vi "Streaming 2945 2955 (FPGA).vi"() -> ()   [LabVIEW 2016]
doc: "Acquires data from the Rx ports and streams the data to the host while receiving data from the host and generating the resulting waveform at the Tx ports of the NI USRP 294x/295x device. Use this VI as a template for the Simple NI-USRP Streaming sample project."
uses:
  <instrlib>/_niInstr/Register Bus/v1/FPGA/Public/Read Cmd Data.ctl
  SubVIs/Stream Control State.ctl
  SubVIs/Rx Parameters.ctl
  HOST/29x5/SubVIs/Start Trigger.ctl
  SubVIs/DDC Parameters.ctl
  <instrlib>/_niInstr/DSP/v1/Shared/Public/IQ Impairments.ctl
  <instrlib>/_niInstr/DSP/v1/Shared/Public/IQ Gain.ctl
  <vilib>/Platform/TimedLoop/XDataNode/timing_clust.ctl
  <vilib>/Platform/TimedLoop/XDataNode/nitl_modes.ctl
  <vilib>/Platform/TimedLoop/XDataNode/wakeup.ctl
  SubVIs/Tx Parameters.ctl
  SubVIs/DUC Parameters.ctl
  <vilib>/rvi/Emulation/niFpgaSctlEmulationGetInTimedLoop.vi
  <vilib>/rvi/Emulation/niFpgaEmulationReportErrorSimple.vi
  <vilib>/rvi/Emulation/niFpgaGetClockAttributes.vi
  <vilib>/rvi/Emulation/niFpgaCriticalErrorInLSC.vi
  <vilib>/rvi/Emulation/niFpgaProcessEmulError.vi
  <vilib>/rvi/Emulation/niFpgaEmulationIsFPGAContextNoSignature.vi
  <vilib>/rvi/DataTransferAndStorage/Container/Common/niFpgaContainerGetUniqueNameForEmu.vi
  <vilib>/rvi/Memory/Memory_Emulation/niFpgaMemoryEmulationCacheClearOnFirstRun.vi
  <vilib>/rvi/Memory/Memory_Emulation/nirvimemoryEmulationManagerCache_MakeExclusive.vi
  <vilib>/rvi/Memory/Memory_Emulation/niFpgaMemoryEmulationValidateCache.vi
  <vilib>/rvi/Memory/Memory_Emulation/nirvimemoryEmulationManagerCache_InsertValue.vi
  <vilib>/Utility/error.llb/Clear Errors.vi
  <vilib>/rvi/Memory/Memory_Emulation/nirvimemoryEmulationManagerCache_ReleaseExclusive.vi
  <vilib>/rvi/Memory/Memory_Emulation/nirvimemoryEmulationManagerCache_GetValue.vi
  <vilib>/rvi/Memory/Memory_Emulation/nirvimemoryEmulationManagerCache_SetValue.vi
  <vilib>/rvi/eio/common/nirviEmuTemplateMethod_errors.vi
  <vilib>/rvi/DataTransferAndStorage/Container/Common/niFpgaContainerExecOnDevCompGetState.vi
  <vilib>/Platform/TimedLoop/XDataNode/XDataNode.xnode
  <vilib>/rvi/DataTransferAndStorage/Container/XNode/niFpgaContainer.xnode
  <vilib>/rvi/DataTransferAndStorage/Register/Emulation/niFpgaRegisterEmulation.vi
  <vilib>/eio/EIONode/EIONode.xnode
  <vilib>/rvi/DataTransferAndStorage/Register/Emulation/niFpgaRegisterEmulationRefIn.vi
  <vilib>/Platform/TimedLoop/XDataNode/XDNodeRunTimeDep.lvlib
  <instrlib>/niUsrpRio/Config/v1/FPGA/niUsrpRio Config v1 FPGA.lvlib
  <instrlib>/_niInstr/DSP/v1/Shared/niInstr DSP v1 Shared.lvlib
  <instrlib>/_niInstr/Instruction Framework/v1/FPGA/Top Level Bus/Register Configuration/Register Configuration.lvclass
  <instrlib>/_niInstr/FIFO Register Bus/v1/FPGA/niInstr FIFO Register Bus v1 FPGA.lvclass
  <instrlib>/_niInstr/Register Bus/v1/FPGA/niInstr Register Bus v1 FPGA.lvlib
panel:
  out "F1":u32
  out "F0":u32
  in  "Simulate Data":bool
  out "fifo reg bus status 1":u32
  out "fifo reg bus data 1":u64
  in  "fifo reg bus ctrl 1":u32
  in  "sfp 0.core reset":bool
  in  "sfp 1.core reset":bool
  out "sfp 0.link reset":bool
  out "sfp 1.link reset":bool
  out "sfp 0.debug info":T1
  out "sfp 1.debug info":T1
  in  "tx 1.led":enum16{"None", "RF 0/TX 1", "RF 1/TX 1"}(ring)
  in  "tx 0.led":enum16{"None", "RF 0/TX 1", "RF 1/TX 1"}(ring)
  in  "rx 0.led":T2(ring)
  in  "rx 1.led":T2(ring)
  in  "rx 2.led":T2(ring)
  in  "rx 3.led":T2(ring)
  in  "tx.data source":enum16{"SFP Port 0", "SFP Port 1", "Host"}(ring)=enum."Host"
  in  "tx.trigger sync enable":bool
  out "tx 1.number of iq data overflows":u64
  out "tx.dsp reset done":bool
  out "tx.state":T3
  out "tx 0.number of iq data overflows":u64
  out "tx.number of fifo underflows":u32
  out "tx.samples processed":u32
  in  "tx.trigger enable":bool
  in  "tx.software trigger":bool
  in  "tx.trigger select":T4=enum."Immediate"
  in  "tx 1.stream enable":bool
  in  "tx 0.stream enable":bool
  in  "tx.samples to generate":u32
  in  "tx.reset":bool=TRUE
  in  "tx.abort":bool
  in  "tx 1.gain":T5={"gain I"=1.0, "gain Q"=1.0}
  in  "tx 1.phase":fxp<+/-,21,0>
  in  "tx 1.frequency shift":fxp<+/-,48,0> format="%#.48g"
  in  "tx 1.impairments":T6={"inline gain I"=0.9999923706054688, "inline gain Q"=0.9999923706054688, "cross gain I"=0.0, "cross gain Q"=0.0, "pre-gain offset I"=0.0, "pre-gain offset Q"=0.0, "post-gain offset I"=0.0, "post-gain offset Q"=0.0}
  in  "tx 0.gain":T5={"gain I"=1.0, "gain Q"=1.0}
  in  "tx 0.impairments":T6={"inline gain I"=0.9999923706054688, "inline gain Q"=0.9999923706054688, "cross gain I"=0.0, "cross gain Q"=0.0, "pre-gain offset I"=0.0, "pre-gain offset Q"=0.0, "post-gain offset I"=0.0, "post-gain offset Q"=0.0}
  in  "tx 0.phase":fxp<+/-,21,0>
  in  "tx 0.frequency shift":fxp<+/-,48,0> format="%#.48g"
  in  "tx.delay":fxp<+/-,18,0>
  in  "tx.input sample rate":fxp<+,48,1>
  out "rx.status":T7={"rx.state"=enum."Idle", "rx.samples processed"=0, "rx.number of fifo overflows"=0, "rx.number of iq data overflows"=[0, 0, 0, 0], "rx.dsp reset done"=FALSE}
  in  "rx 2.stream enable":bool
  in  "rx 3.stream enable":bool
  out "rx 3.number of iq data overflows":u64
  out "rx 2.number of iq data overflows":u64
  in  "rx 3.impairments":T6={"inline gain I"=0.9999923706054688, "inline gain Q"=0.9999923706054688, "cross gain I"=0.0, "cross gain Q"=0.0, "pre-gain offset I"=0.0, "pre-gain offset Q"=0.0, "post-gain offset I"=0.0, "post-gain offset Q"=0.0}
  in  "rx 3.frequency shift":fxp<+/-,48,0> format="%#.48g"
  in  "rx 3.phase":fxp<+/-,21,0>
  in  "rx 2.impairments":T6={"inline gain I"=0.9999923706054688, "inline gain Q"=0.9999923706054688, "cross gain I"=0.0, "cross gain Q"=0.0, "pre-gain offset I"=0.0, "pre-gain offset Q"=0.0, "post-gain offset I"=0.0, "post-gain offset Q"=0.0}
  in  "rx 2.frequency shift":fxp<+/-,48,0> format="%#.48g"
  in  "rx 2.phase":fxp<+/-,21,0>
  in  "RF 1/Tx/Enable":bool
  in  "RF 1/Rx/Enable":bool
  in  "RF 0/Tx/Enable":bool
  in  "RF 0/Rx/Enable":bool
  in  "rx.output sample rate":fxp<+,48,1>
  in  "rx.delay":fxp<+/-,16,0>
  in  "rx 0.frequency shift":fxp<+/-,48,0> format="%#.48g"
  in  "rx 0.phase":fxp<+/-,21,0>
  in  "rx 0.impairments":T6={"inline gain I"=0.9999923706054688, "inline gain Q"=0.9999923706054688, "cross gain I"=0.0, "cross gain Q"=0.0, "pre-gain offset I"=0.0, "pre-gain offset Q"=0.0, "post-gain offset I"=0.0, "post-gain offset Q"=0.0}
  in  "rx 1.impairments":T6={"inline gain I"=0.9999923706054688, "inline gain Q"=0.9999923706054688, "cross gain I"=0.0, "cross gain Q"=0.0, "pre-gain offset I"=0.0, "pre-gain offset Q"=0.0, "post-gain offset I"=0.0, "post-gain offset Q"=0.0}
  in  "rx 1.frequency shift":fxp<+/-,48,0> format="%#.48g"
  in  "rx 1.phase":fxp<+/-,21,0>
  in  "rx.reset":bool=TRUE
  in  "rx.samples to acquire":u32
  in  "rx.abort":bool
  in  "rx 0.stream enable":bool
  in  "rx 1.stream enable":bool
  in  "rx.trigger select":T4=enum."Immediate"
  in  "rx.software trigger":bool
  in  "rx.trigger enable":bool
  out "rx.parameters":T8={"rx.trigger select"=enum."Software", "rx.trigger enable"=FALSE, "rx.trigger sync enable"=FALSE, "rx.stream enable"=[FALSE, FALSE, FALSE, FALSE], "rx.software trigger"=FALSE, "rx.reset"=FALSE, "rx.abort"=FALSE, "rx.samples to acquire"=0, "rx.data sink"=enum."SFP Port 0", "rx.ddc parameters"=[{"output sample rate"=0.0, "delay"=0.0, "frequency shift"=0.0, "impairments"={"inline gain I"=0.0, "inline gain Q"=0.0, "cross gain I"=0.0, "cross gain Q"=0.0, "pre-gain offset I"=0.0, "pre-gain offset Q"=0.0, "post-gain offset I"=0.0, "post-gain offset Q"=0.0}, "phase"=0.0}, {"output sample rate"=0.0, "delay"=0.0, "frequency shift"=0.0, "impairments"={"inline gain I"=0.0, "inline gain Q"=0.0, "cross gain I"=0.0, "cross gain Q"=0.0, "pre-gain offset I"=0.0, "pre-gain offset Q"=0.0, "post-gain offset I"=0.0, "post-gain offset Q"=0.0}, "phase"=0.0}, {"output sample rate"=0.0, "delay"=0.0, "frequency shift"=0.0, "impairments"={"inline gain I"=0.0, "inline gain Q"=0.0, "cross gain I"=0.0, "cross gain Q"=0.0, "pre-gain offset I"=0.0, "pre-gain offset Q"=0.0, "post-gain offset I"=0.0, "post-gain offset Q"=0.0}, "phase"=0.0}, {"output sample rate"=0.0, "delay"=0.0, "frequency shift"=0.0, "impairments"={"inline gain I"=0.0, "inline gain Q"=0.0, "cross gain I"=0.0, "cross gain Q"=0.0, "pre-gain offset I"=0.0, "pre-gain offset Q"=0.0, "post-gain offset I"=0.0, "post-gain offset Q"=0.0}, "phase"=0.0}]} {"rx.ddc parameters"."frequency shift" format="%#.48g"}
  out "rx.samples processed":u32
  out "rx.state":T3
  out "rx 0.number of iq data overflows":u64
  out "rx.number of fifo overflows":u32
  out "rx.dsp reset done":bool
  out "rx 1.number of iq data overflows":u64
  in  "rx.trigger sync enable":bool
  in  "rx.data sink":enum16{"SFP Port 0", "SFP Port 1", "Host"}(ring)=enum."SFP Port 1"
  in  "reg.host read.go rcvd 0":bool
  out "reg.notify host.go 0":bool
  in  "reg.notify host.go rcvd 0":bool
  out "reg.host read.data 0":T10
  in  "reg.reset 0":bool
  # "FPGA utilization"
  # "USRP RIO Simple Streaming FPGA"
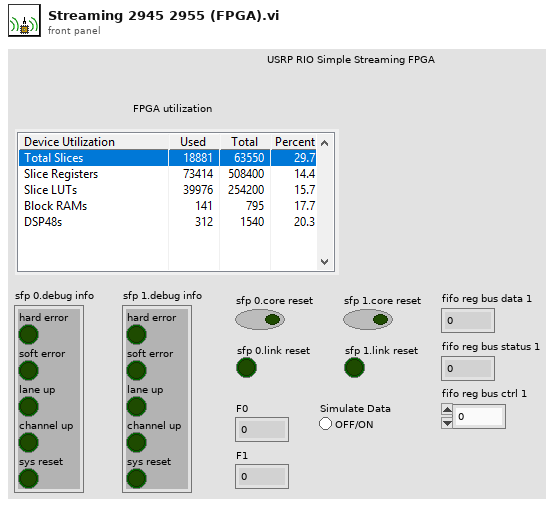
[diagram p1: front panel]
types:
  T1 = cluster{"hard error":bool, "soft error":bool, "lane up":bool, "channel up":bool, "sys reset":bool}
  T2 = enum16{"None", "RF 0/RX 1", "RF 0/RX 2", "RF 1/RX 1", "RF 1/RX 2"}
  T3 = typedef "Stream Control State.ctl" = enum16{"Idle", "Active"}
  T4 = typedef "Start Trigger.ctl" = enum8{"Software", "Digital Edge", "Rx Start Trigger", "Tx Start Trigger", "Immediate", "Future Time Event"}
  T5 = typedef "niInstr DSP v1 Shared.lvlib/IQ Gain.ctl" = cluster{"gain I":fxp<+/-,24,3>, "gain Q":fxp<+/-,24,3>}
  T6 = typedef "niInstr DSP v1 Shared.lvlib/IQ Impairments.ctl" = cluster{"inline gain I":fxp<+/-,18,1>, "inline gain Q":fxp<+/-,18,1>, "cross gain I":fxp<+/-,18,1>, "cross gain Q":fxp<+/-,18,1>, "pre-gain offset I":fxp<+/-,18,1>, "pre-gain offset Q":fxp<+/-,18,1>, "post-gain offset I":fxp<+/-,18,1>, "post-gain offset Q":fxp<+/-,18,1>}
  T7 = cluster{"rx.state":T3, "rx.samples processed":u32, "rx.number of fifo overflows":u32, "rx.number of iq data overflows":u64[], "rx.dsp reset done":bool}
  T8 = typedef "Rx Parameters.ctl" = cluster{"rx.trigger select":T4, "rx.trigger enable":bool, "rx.trigger sync enable":bool, "rx.stream enable":bool[], "rx.software trigger":bool, "rx.reset":bool, "rx.abort":bool, "rx.samples to acquire":u32, "rx.data sink":enum16{"SFP Port 0", "SFP Port 1", "Host"}, "rx.ddc parameters":T9[]}
  T9 = typedef "DDC Parameters.ctl" = cluster{"output sample rate":fxp<+,48,1>, "delay":fxp<+/-,16,0>, "frequency shift":fxp<+/-,48,0>, "impairments":T6, "phase":fxp<+/-,21,0>}
  T10 = typedef "niInstr Register Bus v1 FPGA.lvlib/Read Cmd Data.ctl" = cluster{"go":bool, "data":u32}
  T11 = typedef "XDNodeRunTimeDep.lvlib/timing_clust.ctl" = cluster{"Expected End [f-1]":u64, "Actual End [f-1]":u64, "Finished Late? [f-1]":bool, "Expected End [i-1]":u64, "Actual End [i-1]":u64, "Finished Late? [i-1]":bool, "Expected Start [i]":u64, "Actual Start [i]":u64, "Expected Start [f]":u64, "Actual Start [f]":u64, "Source Name":string, "Structure Name":string, "Period":i64, "Deadline":i64, "Offset":i64, "Start":i64, "Priority":i32, "Timeout":i32, "Mode":T12, "Wakeup Reason":T13, "Error":errorcluster, "Source Type":string, "Secondary Source Type":string, "Global End Time":u64, "Global Start Time":u64, "Frame Duration":u64, "Iteration Duration":u64, "Assigned CPU":i32, "I/O Scan Engine Mode":u32}
  T12 = typedef "XDNodeRunTimeDep.lvlib/nitl_modes.ctl" = enum32{"No Change", "Process missed periods, maintain original phase", "Discard missed periods, maintain original phase", "Process missed periods, ignore original phase", "Discard missed periods, ignore original phase"}
  T13 = typedef "XDNodeRunTimeDep.lvlib/wakeup.ctl" = enum32{"Normal", "Aborted", "Asynchronous wakeup", "Timing source error", "Timed loop error", "Timeout"}
  T14 = cluster{"rx 0.led":enum16{"None", "RF 0/RX 1", "RF 0/RX 2", "RF 1/RX 1", "RF 1/RX 2"}, "rx 1.led":enum16{"None", "RF 0/RX 1", "RF 0/RX 2", "RF 1/RX 1", "RF 1/RX 2"}, "rx 2.led":enum16{"None", "RF 0/RX 1", "RF 0/RX 2", "RF 1/RX 1", "RF 1/RX 2"}, "rx 3.led":enum16{"None", "RF 0/RX 1", "RF 0/RX 2", "RF 1/RX 1", "RF 1/RX 2"}}
  T15 = cluster{"DAC FIFO Reset":refnum<k21>, "RF 0 Rx Swap IQ":refnum<k21>, "RF 0 Rx Negate I":refnum<k21>, "RF 0 Rx Negate Q":refnum<k21>, "RF 0 Rx Data Valid":refnum<k21>, "RF 0 Rx Data Ever Invalid":refnum<k21>, "clear RF 0 Rx Data Ever Invalid":refnum<k21>, "RF 0 Tx Swap IQ":refnum<k21>, "RF 0 Tx Negate I":refnum<k21>, "RF 0 Tx Negate Q":refnum<k21>, "RF 1 Rx Swap IQ":refnum<k21>, "RF 1 Rx Negate I":refnum<k21>, "RF 1 Rx Negate Q":refnum<k21>, "RF 1 Rx Data Valid":refnum<k21>, "RF 1 Rx Data Ever Invalid":refnum<k21>, "clear RF 1 Rx Data Ever Invalid":refnum<k21>, "RF 1 Tx Swap IQ":refnum<k21>, "RF 1 Tx Negate I":refnum<k21>, "RF 1 Tx Negate Q":refnum<k21>}
  T16 = typedef "niUsrpRio Synchronization v1 FPGA.lvlib/Resources.ctl" = cluster{"master":refnum<k21>, "meas.enable":refnum<k21>, "meas.ready":refnum<k21>, "meas.reset":refnum<k21>, "meas.arm":refnum<k21>, "meas.valid":refnum<k21>, "meas.value":refnum<k21>, "meas.oversample factor":refnum<k21>, "cptr":refnum<k21>, "cptr.adjust":refnum<k21>, "cptr.period":refnum<k21>}
  T17 = typedef "niUsrpRio Time v1 FPGA.lvlib/Time Resources.ctl" = cluster{"reset":refnum<k21>, "time":refnum<k21>, "time.previous cptr":refnum<k21>, "new time":refnum<k21>, "new time.when":refnum<k21>, "new time.set":refnum<k21>, "which edge of ref":refnum<k21>, "pps source":refnum<k21>, "internal pps period":refnum<k21>}
  T18 = typedef "niUsrpRio Time v1 FPGA.lvlib/Future Event Resources.ctl" = cluster{"reset":refnum<k21>, "future event.time":refnum<k21>, "future event.ready":refnum<k21>, "future event.set":refnum<k21>, "future event.clear":refnum<k21>, "future event.set in past":refnum<k21>}
  T19 = cluster{"time.resources":T17, "future event.resources":T18, "future event.resources":T18, "future event.resources":T18}
  T20 = cluster{"port clock":refnum<k21>, "TX niInstr AXI4-Stream Reader FXP64x1 v1 FPGA out":refnum<class "niInstr AXI4-Stream Writer FXP64x1 v1 FPGA.lvclass">, "RX niInstr AXI4-Stream Reader FXP64x1 v1 FPGA out":refnum<class "niInstr AXI4-Stream Reader FXP64x1 v1 FPGA.lvclass">, "Port 0 Debug CLIP Resources":cluster{"Hard Error":refnum<k21>, "Soft Error":refnum<k21>, "Lane Up":refnum<k21>, "Channel Up":refnum<k21>, "Sys Reset":refnum<k21>}, "debug info":refnum<k21>}
  T21 = cluster{"port clock":refnum<k21>, "TX niInstr AXI4-Stream Reader FXP64x1 v1 FPGA out":refnum<class "niInstr AXI4-Stream Writer FXP64x1 v1 FPGA.lvclass">, "RX niInstr AXI4-Stream Reader FXP64x1 v1 FPGA out":refnum<class "niInstr AXI4-Stream Reader FXP64x1 v1 FPGA.lvclass">, "Port 1 Debug CLIP Resources":cluster{"Hard Error":refnum<k21>, "Soft Error":refnum<k21>, "Lane Up":refnum<k21>, "Channel Up":refnum<k21>, "Sys Reset":refnum<k21>}, "debug info":refnum<k21>}
  T22 = cluster{"rx.trigger select":T4, "rx.trigger enable":bool, "rx.trigger sync enable":bool, bool[], "rx.software trigger":bool, "rx.reset":bool, "rx.abort":bool, "rx.samples to acquire":u32, "rx.data sink":enum16{"SFP Port 0", "SFP Port 1", "Host"}, T9[]}
  T23 = typedef "Clock Cross Resources.ctl" = cluster{"register instruction":refnum<k21>, "read completion":refnum<k21>}
  T24 = typedef "niInstr Register Bus v1 FPGA.lvlib/Register Instruction.ctl" = cluster{"subsystem":u8, "address":u16, "data":u32, "valid":bool, "read":bool}
  T25 = typedef "niInstr Register Bus v1 FPGA.lvlib/Read Completion.ctl" = cluster{"data":u32, "valid":bool}
  T26 = typedef "Tx Parameters.ctl" = cluster{"tx.trigger select":T4, "tx.trigger enable":bool, "tx.trigger sync enable":bool, "tx.stream enable":bool[], "tx.software trigger":bool, "tx.reset":bool, "tx.abort":bool, "tx.samples to generate":u32, "tx.data source":enum16{"SFP Port 0", "SFP Port 1", "Host"}, "tx.duc parameters":T27[]}
  T27 = typedef "DUC Parameters.ctl" = cluster{"frequency shift":fxp<+/-,48,0>, "impairments":T6, "phase":fxp<+/-,21,0>, "input sample rate":fxp<+,48,1>, "gain":T5, "delay":fxp<+/-,18,0>}
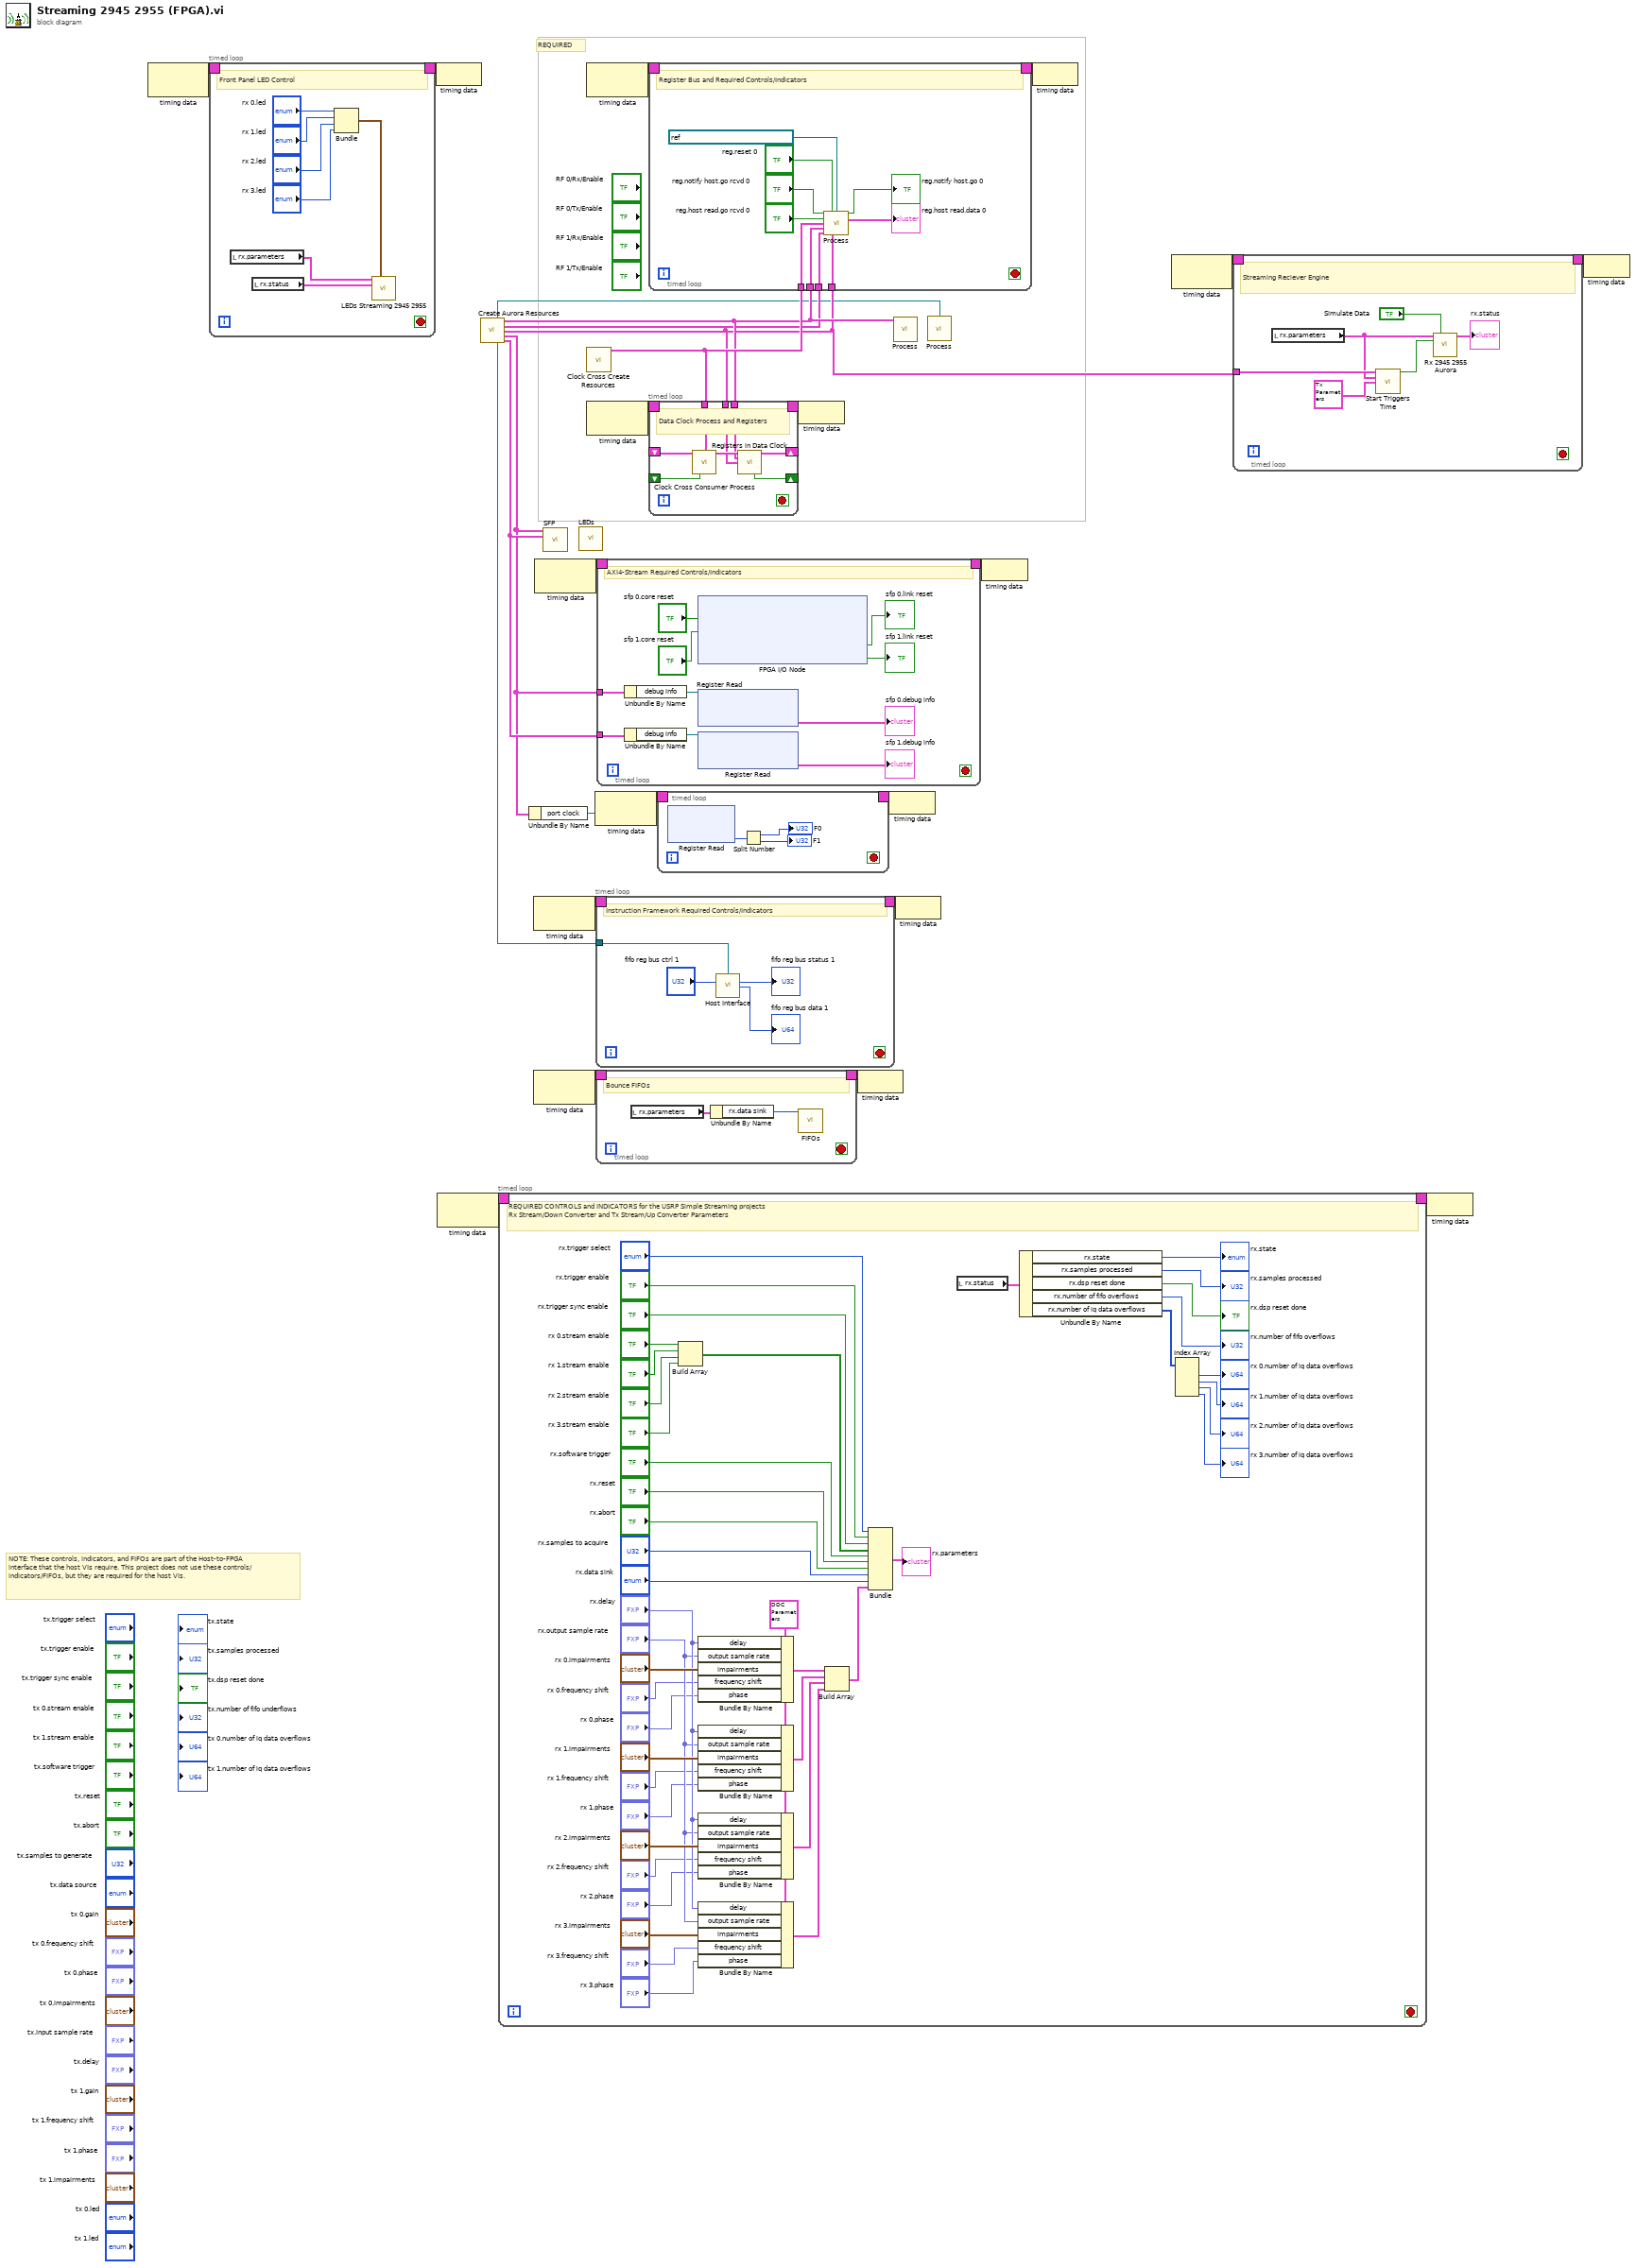
[diagram p0: block diagram]
diagram:
  # "NOTE: These controls, indicators, and FIFOs are part of the Host-to-FPGA interface that the host VIs require. This project does not use these controls/indicators/FIFOs, but they are required for the host VIs."
  # "REQUIRED"
  n1 = node-c288() -> (w18:T11)  [unwired: 1 in]
  n2 = timed-loop {
    timing: w18 -> [_]
    timing-out: [_] -> w17
    stop <- _ stop-if-true
    # "Front Panel LED Control"
    n3 = local read "rx.parameters"() -> (w29:T8)
    n4 = local read "rx.status"() -> (w28:T7)
    n5 = Bundle("rx 0.led"="rx 0.led", "rx 1.led"="rx 1.led", "rx 2.led"="rx 2.led", "rx 3.led"="rx 3.led") -> (w30:T14)  [unwired: 1 in]
    n6 = call "LEDs Streaming 2945 2955.vi"("rx.parameters"=w29, "rx.leds"=w30, "rx.status"=w28) -> ()  [unwired: 13 in]
  }
  n7 = node-c288(w17) -> ()
  n8 = node-c288() -> (w23:T11)  [unwired: 1 in]
  n9 = call "Create Aurora Resources.vi"() -> ("framework.resources"=w13:refnum<class "Register Configuration.lvclass">, "config.resources"=w16:T15, "sync.resources"=w15:T16, "time.resources"=w14:T19, "sfp 0.resources"=w2:T20, "producer.resources"=w8:refnum<class "niInstr FIFO Register Bus v1 FPGA.lvclass">, "sfp 1.resources"=w5:T21)  [unwired: 9 in]
  n10 = timed-loop {
    timing: w23 -> [_]
    timing-out: [_] -> w22
    stop <- _ stop-if-true
    w63 = T9 {"output sample rate"=1.0, "delay"=0.0, "frequency shift"=0.0, "impairments"={"inline gain I"=0.9999923706054688, "inline gain Q"=0.9999923706054688, "cross gain I"=0.0, "cross gain Q"=0.0, "pre-gain offset I"=0.0, "pre-gain offset Q"=0.0, "post-gain offset I"=0.0, "post-gain offset Q"=0.0}, "phase"=0.0} ("DDC Parameters")
    # "REQUIRED CONTROLS and INDICATORS for the USRP Simple Streaming projects\nRx Stream/Down Converter and Tx Stream/Up Converter Parameters"
    n11 = Build Array("rx 0.stream enable", "rx 1.stream enable", "rx 2.stream enable", "rx 3.stream enable") -> (w44:bool[])
    n12 = Bundle By Name(cluster=w63, "delay"="rx.delay", "output sample rate"="rx.output sample rate", "impairments"="rx 0.impairments", "frequency shift"="rx 0.frequency shift", "phase"="rx 0.phase") -> (w79:T9)
    n13 = Bundle By Name(cluster=w63, "delay"="rx.delay", "output sample rate"="rx.output sample rate", "impairments"="rx 1.impairments", "frequency shift"="rx 1.frequency shift", "phase"="rx 1.phase") -> (w80:T9)
    n14 = Bundle By Name(cluster=w63, "delay"="rx.delay", "output sample rate"="rx.output sample rate", "impairments"="rx 2.impairments", "frequency shift"="rx 2.frequency shift", "phase"="rx 2.phase") -> (w60:T9)
    n15 = Bundle By Name(cluster=w63, "delay"="rx.delay", "output sample rate"="rx.output sample rate", "impairments"="rx 3.impairments", "frequency shift"="rx 3.frequency shift", "phase"="rx 3.phase") -> (w59:T9)
    n16 = Build Array(w79, w80, w60, w59) -> (w70:T9[])
    n17 = Bundle("rx.trigger select"="rx.trigger select", "rx.trigger enable"="rx.trigger enable", "rx.trigger sync enable"="rx.trigger sync enable", w44, "rx.software trigger"="rx.software trigger", "rx.reset"="rx.reset", "rx.abort"="rx.abort", "rx.samples to acquire"="rx.samples to acquire", "rx.data sink"="rx.data sink", w70) -> (→"rx.parameters":T22)  [unwired: 1 in]
    n18 = local read "rx.status"() -> (w69:T7)
    n19 = Unbundle By Name(w69) -> ("rx.state"=→"rx.state":T3, "rx.samples processed"=→"rx.samples processed":u32, "rx.dsp reset done"=→"rx.dsp reset done":bool, "rx.number of fifo overflows"=→"rx.number of fifo overflows":u32, "rx.number of iq data overflows"=w41:u64[])
    n20 = Index Array(array=w41) -> (element #1=→"rx 0.number of iq data overflows":u64, element #2=→"rx 1.number of iq data overflows":u64, element #3=→"rx 2.number of iq data overflows":u64, element #4=→"rx 3.number of iq data overflows":u64)  [unwired: 4 in]
  }
  n21 = Unbundle By Name(w2) -> ("port clock"=w1:refnum<k21>)
  n22 = node-c288() -> (w10:T11)  [unwired: 1 in]
  n23 = node-c288() -> (w7:T11)  [unwired: 1 in]
  n24 = node-c288() -> (w12:T11)  [unwired: 1 in]
  n25 = call "SFP.vi"("sfp 0.resources"=w2, "sfp 1.resources"=w5) -> ()  [unwired: 14 in]
  n26 = call "LEDs.vi"() -> ()  [unwired: 1 in]
  n27 = node-c288() -> (w27:T11)  [unwired: 1 in]
  n28 = call "Clock Cross Create Resources.vi"() -> ("resources"=w19:T23)  [unwired: 15 in]
  n29 = node-c288() -> (w21:T11)  [unwired: 1 in]
  n30 = node-c288(w1) -> (w4:T11)
  n31 = timed-loop {
    timing: w10 -> [_]
    timing-out: [_] -> w9
    tunnel: w8 -> [w86]
    stop <- _ stop-if-true
    # "Instruction Framework Required Controls/Indicators"
    n32 = call <instrlib>:"Host Interface.vi"("fifo register bus"=w86, "fifo reg bus ctrl 0"="fifo reg bus ctrl 1") -> ("fifo reg bus status 0"=→"fifo reg bus status 1":u32, "fifo reg bus data 0"=→"fifo reg bus data 1":u64)  [unwired: 12 in]
  }
  n33 = timed-loop {
    timing: w7 -> [_]
    timing-out: [_] -> w6
    stop <- _ stop-if-true
    # "Bounce FIFOs"
    n34 = local read "rx.parameters"() -> (w90:T8)
    n35 = Unbundle By Name(w90) -> ("rx.data sink"=w89:enum16{"SFP Port 0", "SFP Port 1", "Host"})
    n36 = call "FIFOs.vi"("rx.data sink"=w89) -> ()  [unwired: 15 in]
  }
  n37 = timed-loop {
    timing: w12 -> [_]
    timing-out: [_] -> w11
    tunnel: w2 -> [w98]
    tunnel: w5 -> [w97]
    stop <- _ stop-if-true
    # "AXI4-Stream Required Controls/Indicators"
    n38 = Unbundle By Name(w98) -> ("debug info"=w96:refnum<k21>)
    n39 = Unbundle By Name(w97) -> ("debug info"=w95:refnum<k21>)
    n40 = xnode "FPGA I/O Node"("MGT Socket\\dPort0CoreReset"="sfp 0.core reset", "MGT Socket\\dPort1CoreReset"="sfp 1.core reset") -> ("MGT Socket\\dPort0LinkResetOut"=→"sfp 0.link reset":bool, "MGT Socket\\dPort1LinkResetOut"=→"sfp 1.link reset":bool)  [unwired: 4 in, 4 out]
    n41 = xnode ("Register Read")("Register In"=w96) -> ("Data"=→"sfp 0.debug info":T1)  [unwired: 1 out]
    n42 = xnode ("Register Read")("Register In"=w95) -> ("Data"=→"sfp 1.debug info":T1)  [unwired: 1 out]
  }
  n43 = timed-loop "Register Bus and Required Controls/Indicators" {
    timing: w27 -> [_]
    timing-out: [_] -> w26
    tunnel: w16 -> [w107]
    tunnel: w15 -> [w106]
    tunnel: w14 -> [w105]
    tunnel: w19 -> [w108]
    stop <- _ stop-if-true
    # "Register Bus and Required Controls/Indicators"
    n44 = call <instrlib>:"Process.vi"("reg.notify host.go rcvd"="reg.notify host.go rcvd 0", "reg.reset"="reg.reset 0", "reg.instruction fifo"=refnum<k21> "reg.host instruction fifo 0" ("reg.host instruction fifo"), "reg.host read.go rcvd"="reg.host read.go rcvd 0", "clock cross resources"=w108, "config.resources"=w107, "sync.resources"=w106, "time.resources"=w105) -> ("reg.notify host.go"=→"reg.notify host.go 0":bool, "reg.host read.data"=→"reg.host read.data 0":T10)  [unwired: 6 in]
  }
  n45 = timed-loop {
    timing: w21 -> [_]
    timing-out: [_] -> w20
    shift-right: [w123] -> _
    shift-left: _ -> [w120]
    shift-right: [w122] -> _
    shift-left: _ -> [w121]
    tunnel: w16 -> [w119]
    tunnel: w19 -> [w118]
    tunnel: w14 -> [w117]
    stop <- _ stop-if-true
    # "Data Clock Process and Registers"
    n46 = call "Clock Cross Consumer Process.vi"("read completion"=w120, "resources"=w118, "ready for output"=w121) -> ("register instruction"=w124:T24)  [unwired: 12 in]
    n47 = call "Registers in Data Clock.vi"("register instruction"=w124, "config.resources"=w119, "time.resources"=w117) -> ("read completion out"=w123:T25, "ready for input"=w122:bool)  [unwired: 11 in]
  }
  n48 = timed-loop {
    timing: w4 -> [_]
    timing-out: [_] -> w3
    stop <- _ stop-if-true
    n49 = xnode ("Register Read")() -> ("Data"=w129:u64)  [unwired: 1 in, 1 out]
    n50 = Split Number(x=w129) -> (hi(x)=→"F0":u32, lo(x)=→"F1":u32)
  }
  n51 = node-c288(w20) -> ()
  n52 = node-c288(w6) -> ()
  n53 = node-c288(w3) -> ()
  n54 = call <instrlib>:"Process.vi"("resources"=w16) -> ()  [unwired: 15 in]
  n55 = node-c288(w9) -> ()
  n56 = call <instrlib>:"Process.vi"("register configuration"=w13) -> ()  [unwired: 15 in]
  n57 = node-c288(w11) -> ()
  n58 = node-c288(w26) -> ()
  n59 = node-c288() -> (w25:T11)  [unwired: 1 in]
  n60 = timed-loop "Streaming Transceiver Engine" {
    timing: w25 -> [_]
    timing-out: [_] -> w24
    tunnel: w14 -> [w136]
    stop <- _ stop-if-true
    # "Streaming Reciever Engine"
    n61 = local read "rx.parameters"() -> (w135:T8)
    n62 = call "Start Triggers Time.vi"("time.resources"=w136, "rx.parameters"=w135, "tx.parameters"=T26 {"tx.trigger select"=enum."Software", "tx.trigger enable"=FALSE, "tx.trigger sync enable"=FALSE, "tx.stream enable"=[FALSE, FALSE], "tx.software trigger"=FALSE, "tx.reset"=FALSE, "tx.abort"=FALSE, "tx.samples to generate"=0, "tx.data source"=enum."SFP Port 0", "tx.duc parameters"=[{"frequency shift"=0.0, "impairments"={"inline gain I"=0.0, "inline gain Q"=0.0, "cross gain I"=0.0, "cross gain Q"=0.0, "pre-gain offset I"=0.0, "pre-gain offset Q"=0.0, "post-gain offset I"=0.0, "post-gain offset Q"=0.0}, "phase"=0.0, "input sample rate"=0.0, "gain"={"gain I"=0.0, "gain Q"=0.0}, "delay"=0.0}, {"frequency shift"=0.0, "impairments"={"inline gain I"=0.0, "inline gain Q"=0.0, "cross gain I"=0.0, "cross gain Q"=0.0, "pre-gain offset I"=0.0, "pre-gain offset Q"=0.0, "post-gain offset I"=0.0, "post-gain offset Q"=0.0}, "phase"=0.0, "input sample rate"=0.0, "gain"={"gain I"=0.0, "gain Q"=0.0}, "delay"=0.0}]}) -> ("rx.start trigger"=w137:bool)  [unwired: 11 in, 1 out]
    n63 = call "Rx 2945 2955 Aurora.vi"("rx.parameters"=w135, "Simulate Data"="Simulate Data", "rx.start trigger"=w137) -> ("rx.status"=→"rx.status":T7)  [unwired: 12 in]
  }
  n64 = node-c288(w22) -> ()
  n65 = node-c288(w24) -> ()
